vi "Actor Core.vi"(8 "error in":errorcluster, 11 "TRExperimentsRaw in":refnum<class "Solutions.lvclass">) -> (0 "error out":errorcluster, 3 "Actor out":refnum<class "Actor.lvclass">)   [LabVIEW 2020, in "Forms.lvlib" / "Solutions.lvclass"]
doc: "The user interface for this panel.\n\n----\nPlease see the following web address for additional documentation and tutorial information:\nhttp://www.mooregoodideas.com/mgi-panel-manager/\n\nAuthor: Derek Trepanier\n\nCopyright (c) 2018, Moore Good Ideas, Inc.\n\nAll rights reserved.\n\nRedistribution and use in source and binary forms, with or without modification, are permitted provided that the following conditions are met:\n\n * Redistributions of source code must retain the above copyright notice, this list of conditions and the following disclaimer.\n * Redistributions in binary form must reproduce the above copyright notice, this list of conditions and the following disclaimer in the documentation and/or other materials provided with the distribution.\n * Neither the name of Moore Good Ideas, Inc. nor the names of its contributors may be used to endorse or promote products derived from this software without specific prior written permission.\n\nTHIS SOFTWARE IS PROVIDED BY THE COPYRIGHT HOLDERS AND CONTRIBUTORS \"AS IS\" AND ANY EXPRESS OR IMPLIED WARRANTIES, INCLUDING, BUT NOT LIMITED TO, THE IMPLIED WARRANTIES OF MERCHANTABILITY AND FITNESS FOR A PARTICULAR PURPOSE ARE DISCLAIMED. IN NO EVENT SHALL THE COPYRIGHT OWNER OR CONTRIBUTORS BE LIABLE FOR ANY DIRECT, INDIRECT, INCIDENTAL, SPECIAL, EXEMPLARY, OR CONSEQUENTIAL DAMAGES (INCLUDING, BUT NOT LIMITED TO, PROCUREMENT OF SUBSTITUTE GOODS OR SERVICES; LOSS OF USE, DATA, OR PROFITS; OR BUSINESS INTERRUPTION) HOWEVER CAUSED AND ON ANY THEORY OF LIABILITY, WHETHER IN CONTRACT, STRICT LIABILITY, OR TORT (INCLUDING NEGLIGENCE OR OTHERWISE) ARISING IN ANY WAY OUT OF THE USE OF THIS SOFTWARE, EVEN IF ADVISED OF THE POSSIBILITY OF SUCH DAMAGE."
uses:
  Solutions.lvclass
  C:/Users/User/Desktop/Raman Program/Database OOP/source/Forms AF/Form Controller/Panel Form Controller.lvclass
  <vilib>/ActorFramework/Actor/Actor.lvclass
  Database OOP/Field/Text Field Info.ctl
  Database OOP/Field/Numeric Field Info.ctl
  Database OOP/Open Form Button/Open Form Button Class/Open Form.lvclass
  C:/Users/User/Desktop/Raman Program/Database OOP/source/Database OOP/Button/Button Class/Button.lvclass
  Form Controller/Panel Form Controller.lvclass/Panel Form Controller.ctl
  Database OOP/Field/Field Class/Constructor by Info Cluster Text.vi
  Database OOP/Field/Field Class/Constructor by Info Cluster Numeric.vi
  Form Controller/Panel Form Controller.lvclass
  Database OOP/Field.lvlib
  Database OOP/Field/Field Class/Field.lvclass
panel:
  in  "Cation (mM)":dbl
  in  "pH":dbl
  in  "Cation":string
  in  "Anion":string
  in  "Display Name":string
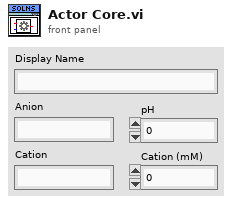
[diagram p1: front panel]
types:
  T1 = typedef "Panel Form Controller.lvlib/Builder Cluster.ctl" = cluster{"Field Map":map{string, refnum<class "Field.lvclass">}, "Button Map":map{string, refnum<class "Button.lvclass">}, "Initialized Field":refnum<class "Field.lvclass">, "VI Ctrl Array":refnum<vi>[]}
  T2 = typedef "Field.lvlib/Text Field Info.ctl" = cluster{"Ctl Refnum":refnum<vi>, "Table":string, "Column":string}
  T3 = typedef "Field.lvlib/Numeric Field Info.ctl" = cluster{"Ctl Refnum":refnum<vi>, "Table":string, "Column":string}
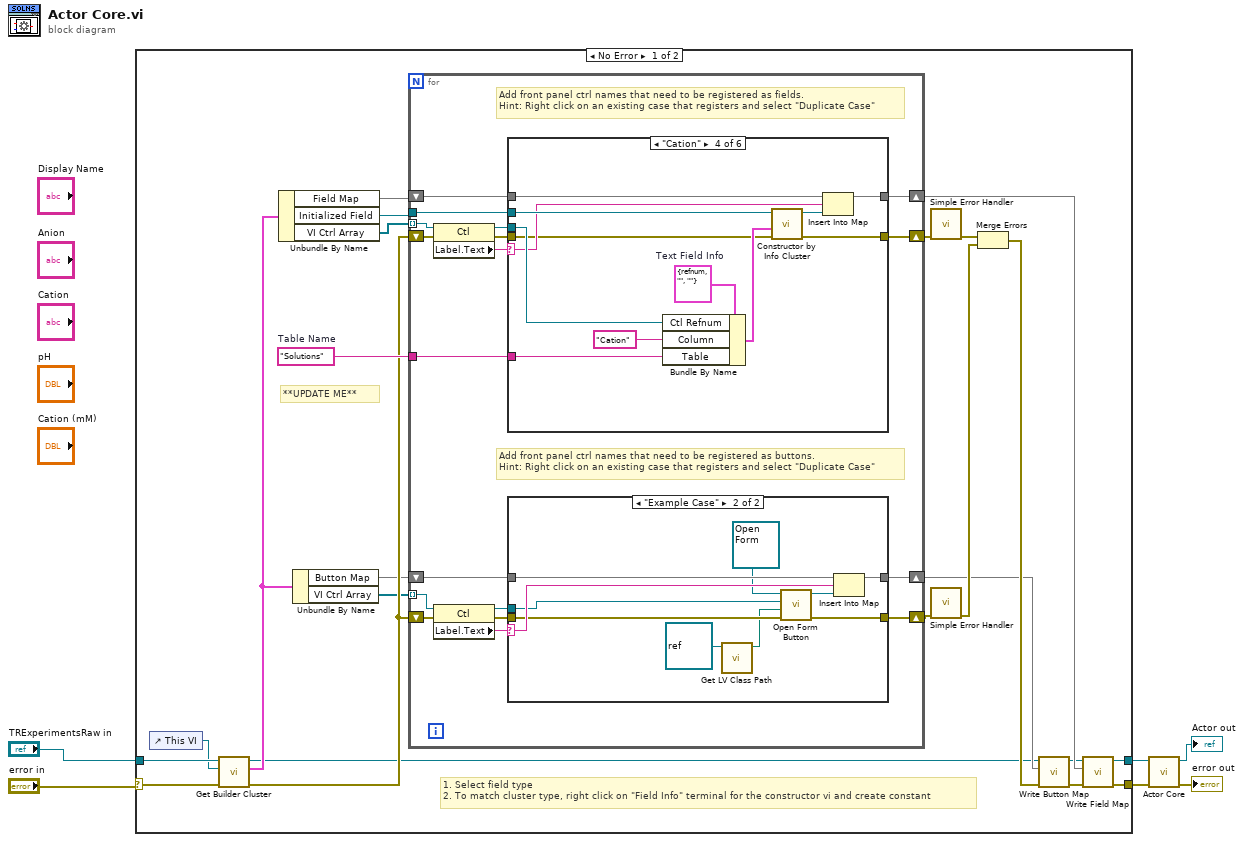
[diagram p0: block diagram]
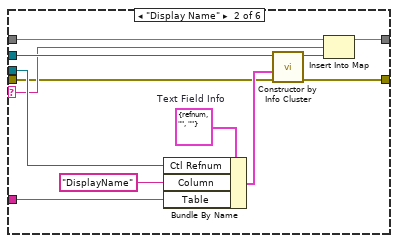
[diagram p4: hidden frame]
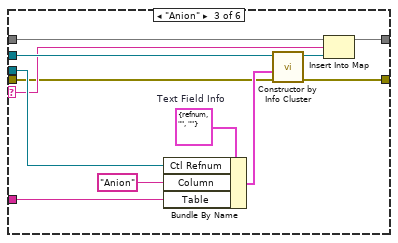
[diagram p5: hidden frame]
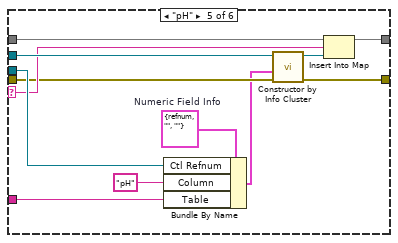
[diagram p6: hidden frame]
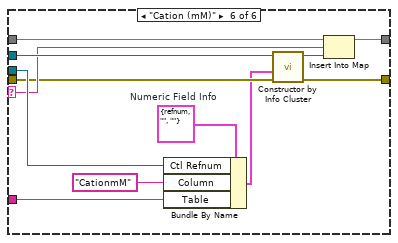
[diagram p7: hidden frame]
diagram:
  n1 = case shown="No Error" "error in" {
    selector: "error in" -> [w10 w123]
    tunnel: "TRExperimentsRaw in" -> [w27 w122]
    tunnel: [w9 w123] -> w3
    tunnel: [w8 w122] -> w4
    frame No Error {
      w29 = "Solutions"  # Table Name
      # "1. Select field type\n2. To match cluster type, right click on \"Field Info\" terminal for the constructor vi and create constant"
      # "**UPDATE ME**"
      n2 = control-ref of="This VI"() -> (w7:refnum<vi>)
      n3 = call "Get Builder Cluster.vi"("error in (no error)"=w10, "VI Refnum"=w7, "Panel Form Controller in"=w27) -> ("error out"=w22:errorcluster, "Builder Cluster"=w20:T1, "Panel Form Controller out"=w11:refnum<class "Solutions.lvclass">)  [unwired: 6 in]
      n4 = Unbundle By Name(w20) -> ("Field Map"=w26:map{string, refnum<class "Field.lvclass">}, "Initialized Field"=w25:refnum<class "Field.lvclass">, "VI Ctrl Array"=w24:refnum<vi>[])
      n5 = Unbundle By Name(w20) -> ("Button Map"=w19:map{string, refnum<class "Button.lvclass">}, "VI Ctrl Array"=w18:refnum<vi>[])
      n6 = for {
        tunnel: w24 -> [w47] mode=indexing
        tunnel: w25 -> [w45]
        tunnel: w29 -> [w44]
        shift-right: [w38] -> w23
        shift-left: w26 -> [w39]
        shift-right: [w43] -> w28
        shift-left: w22 -> [w42]
        shift-right: [w37] -> w21
        shift-left: w22 -> [w36]
        tunnel: w18 -> [w34] mode=indexing
        shift-right: [w31] -> w12
        shift-left: w19 -> [w32]
        # "Add front panel ctrl names that need to be registered as buttons.\nHint: Right click on an existing case that registers and select \"Duplicate Case\""
        # "Add front panel ctrl names that need to be registered as fields.\nHint: Right click on an existing case that registers and select \"Duplicate Case\""
        n7 = property class="Ctl"(reference=w47, error in=w42) -> (reference out=w46:refnum<vi>, error out=w41:errorcluster, "Label.Text"=w40:string)
        n8 = property class="Ctl"(reference=w34, error in=w36) -> (reference out=w33:refnum<vi>, error out=w35:errorcluster, "Label.Text"=w30:string)
        n9 = case shown="\"Cation\"" w40 {
          selector: w40 -> [_ w65 w77 w89 w103 w115]
          tunnel: w46 -> [_ w70 w82 w94 w108 w120]
          tunnel: w45 -> [_ w73 w85 w97 w109 w121]
          tunnel: w44 -> [_ w69 w81 w93 w107 w119]
          tunnel: w39 -> [w61 w68 w80 w92 w106 w118]
          tunnel: [w61 w67 w79 w91 w105 w117] -> w38
          tunnel: [w60 w64 w76 w88 w102 w114] -> w43
          tunnel: w41 -> [w60 w63 w75 w87 w101 w113]
          frame Default {
          }
          frame "Display Name" {
            w72 = T2 {"Ctl Refnum"=refnum, "Table"="", "Column"=""}  # Text Field Info
            n10 = Bundle By Name(cluster=w72, "Ctl Refnum"=w70, "Column"="DisplayName", "Table"=w69) -> (w71:T2)
            n11 = call-poly "Constructor by Info Cluster.vi"("error in (no error)"=w63, "Text Field Info"=w71, "Field in"=w73) -> ("error out"=w64:errorcluster, "Field out"=w66:refnum<class "Field.lvclass">)  [unwired: 7 in]
            n12 = Insert Into Map(map in=w68, key=w65, value=w66) -> (map out=w67:map{string, refnum<class "Field.lvclass">})  [unwired: 2 out]
          }
          frame "Anion" {
            w84 = T2 {"Ctl Refnum"=refnum, "Table"="", "Column"=""}  # Text Field Info
            n13 = Bundle By Name(cluster=w84, "Ctl Refnum"=w82, "Column"="Anion", "Table"=w81) -> (w83:T2)
            n14 = call-poly "Constructor by Info Cluster.vi"("error in (no error)"=w75, "Text Field Info"=w83, "Field in"=w85) -> ("error out"=w76:errorcluster, "Field out"=w78:refnum<class "Field.lvclass">)  [unwired: 7 in]
            n15 = Insert Into Map(map in=w80, key=w77, value=w78) -> (map out=w79:map{string, refnum<class "Field.lvclass">})  [unwired: 2 out]
          }
          frame "Cation" {
            w96 = T2 {"Ctl Refnum"=refnum, "Table"="", "Column"=""}  # Text Field Info
            n16 = Bundle By Name(cluster=w96, "Ctl Refnum"=w94, "Column"="Cation", "Table"=w93) -> (w95:T2)
            n17 = call-poly "Constructor by Info Cluster.vi"("error in (no error)"=w87, "Text Field Info"=w95, "Field in"=w97) -> ("error out"=w88:errorcluster, "Field out"=w90:refnum<class "Field.lvclass">)  [unwired: 7 in]
            n18 = Insert Into Map(map in=w92, key=w89, value=w90) -> (map out=w91:map{string, refnum<class "Field.lvclass">})  [unwired: 2 out]
          }
          frame "pH" {
            w99 = T3 {"Ctl Refnum"=refnum, "Table"="", "Column"=""}  # Numeric Field Info
            n19 = Bundle By Name(cluster=w99, "Ctl Refnum"=w108, "Column"="pH", "Table"=w107) -> (w98:T3)
            n20 = call-poly "Constructor by Info Cluster.vi"("error in (no error)"=w101, "Numeric Field Info"=w98, "Field in"=w109) -> ("error out"=w102:errorcluster, "Field out"=w104:refnum<class "Field.lvclass">)  [unwired: 7 in]
            n21 = Insert Into Map(map in=w106, key=w103, value=w104) -> (map out=w105:map{string, refnum<class "Field.lvclass">})  [unwired: 2 out]
          }
          frame "Cation (mM)" {
            w111 = T3 {"Ctl Refnum"=refnum, "Table"="", "Column"=""}  # Numeric Field Info
            n22 = Bundle By Name(cluster=w111, "Ctl Refnum"=w120, "Column"="CationmM", "Table"=w119) -> (w110:T3)
            n23 = call-poly "Constructor by Info Cluster.vi"("error in (no error)"=w113, "Numeric Field Info"=w110, "Field in"=w121) -> ("error out"=w114:errorcluster, "Field out"=w116:refnum<class "Field.lvclass">)  [unwired: 7 in]
            n24 = Insert Into Map(map in=w118, key=w115, value=w116) -> (map out=w117:map{string, refnum<class "Field.lvclass">})  [unwired: 2 out]
          }
        }
        n25 = case shown="\"Example Case\"" w30 {
          selector: w30 -> [_ w57]
          tunnel: w33 -> [_ w55]
          tunnel: [w49 w53] -> w37
          tunnel: w35 -> [w49 w54]
          tunnel: w32 -> [w48 w59]
          tunnel: [w48 w58] -> w31
          frame Default {
          }
          frame "Example Case" {
            n26 = call <vilib>:"Get LV Class Path.vi"("object"=refnum<class> refnum) -> ("class path"=w51:path)  [unwired: 9 in, 1 out]
            n27 = call "Open Form Button.vi"("error in (no error)"=w54, "Class Path"=w51, "Ctl Refnum"=w55, "Open Form in"=refnum<class "Open Form.lvclass"> refnum) -> ("error out"=w53:errorcluster, "Open Form out"=w56:refnum<class "Open Form.lvclass">)  [unwired: 6 in]
            n28 = Insert Into Map(map in=w59, key=w57, value=w56) -> (map out=w58:map{string, refnum<class "Button.lvclass">})  [unwired: 2 out]
          }
        }
      }
      n29 = call <vilib>:"Simple Error Handler.vi"("error in (no error)"=w28) -> ("error out"=w16:errorcluster)  [unwired: 4 in, 4 out]
      n30 = call <vilib>:"Simple Error Handler.vi"("error in (no error)"=w21) -> ("error out"=w17:errorcluster)  [unwired: 4 in, 4 out]
      n31 = Merge Errors(w16, w17) -> (w15:errorcluster)
      n32 = call "Write Button Map.vi"("error in (no error)"=w15, "Button Map"=w12, "Panel Form Controller in"=w11) -> ("error out"=w14:errorcluster, "Panel Form Controller out"=w13:refnum<class "Solutions.lvclass">)  [unwired: 7 in]
      n33 = call "Write Field Map.vi"("error in (no error)"=w14, "Field Map"=w23, "Panel Form Controller in"=w13) -> ("error out"=w9:errorcluster, "Panel Form Controller out"=w8:refnum<class "Solutions.lvclass">)  [unwired: 7 in]
    }
    frame Error {
    }
  }
  n34 = call-parent "Actor Core.vi"("error in"=w3, "Panel Form Controller in"=w4) -> ("error out"=→"error out":errorcluster, "Actor out"=→"Actor out":refnum<class "Actor.lvclass">)  [unwired: 8 in]
